vi "Close.vi"(6 "deadline":T1={"mode"=enum."Relative", "deadline (ms)"=30000}, 8 "error in (no error)":errorcluster, 11 "subprocess in":refnum<class "Buffered Subprocess.lvclass">) -> (0 "error out":errorcluster, 2 "return code":u8, 3 "subprocess out":refnum<class "Buffered Subprocess.lvclass">, 5 "stderr remaining":u8[](array[numeric]), 7 "stdout remaining":u8[](array[numeric]))   [LabVIEW 2020, in "NI_Subprocess.lvlib" / "Buffered Subprocess.lvclass"]
uses:
  <vilib>/Subprocess/Buffered Subprocess/Buffered Subprocess.lvclass
  <vilib>/Utility/Deadline/Deadline.ctl
  <vilib>/Utility/Deadline/Mode.ctl
  <vilib>/Subprocess/Buffered Subprocess/Buffered Subprocess.lvclass/Buffered Subprocess.ctl
  <vilib>/Subprocess/Subprocess/Subprocess.lvclass
  <vilib>/Array/Bytestream/Bytestream.lvclass
  <vilib>/Utility/Deadline/NI_Deadline.lvlib
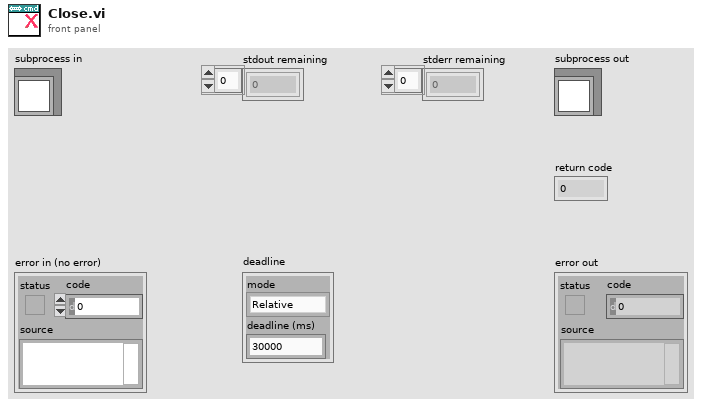
[diagram p1: front panel]
types:
  T1 = typedef "NI_Deadline.lvlib/Deadline.ctl" = cluster{"mode":T2, "deadline (ms)":u32}
  T2 = typedef "NI_Deadline.lvlib/Mode.ctl" = enum16{"Relative", "Use deadline", "Wait forever", "Nonblocking", "N/A"}
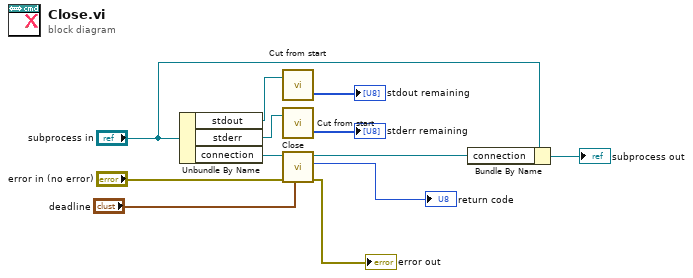
[diagram p0: block diagram]
diagram:
  n1 = Unbundle By Name("subprocess in") -> ("stdout"=w7:refnum<class "Bytestream.lvclass">, "stderr"=w8:refnum<class "Bytestream.lvclass">, "connection"=w6:refnum<class "Subprocess.lvclass">)
  n2 = call <vilib>:"Cut from start.vi"("bytestream in"=w7) -> ("data"=→"stdout remaining":u8[])  [unwired: 1 in, 1 out]
  n3 = call <vilib>:"Cut from start.vi"("bytestream in"=w8) -> ("data"=→"stderr remaining":u8[])  [unwired: 1 in, 1 out]
  n4 = call <vilib>:"Close.vi"("deadline"="deadline", "error in (no error)"="error in (no error)", "subprocess in"=w6) -> ("error out"=→"error out":errorcluster, "return code"=→"return code":u8, "subprocess out"=w4:refnum<class "Subprocess.lvclass">)  [unwired: 6 in]
  n5 = Bundle By Name(cluster="subprocess in", "connection"=w4) -> (→"subprocess out":refnum<class "Buffered Subprocess.lvclass">)
